vi "Dequeue Message.vi"(8 "error in (no error)":errorcluster, 10 "queue in":refnum<queue>) -> (0 "error out":errorcluster, 2 "queue out":refnum<queue>, 3 "Message out":refnum<class "Message.lvclass">)   [LabVIEW 2021, in "Architecture.lvlib" / "Message.lvclass"]
uses:
  Message.lvclass
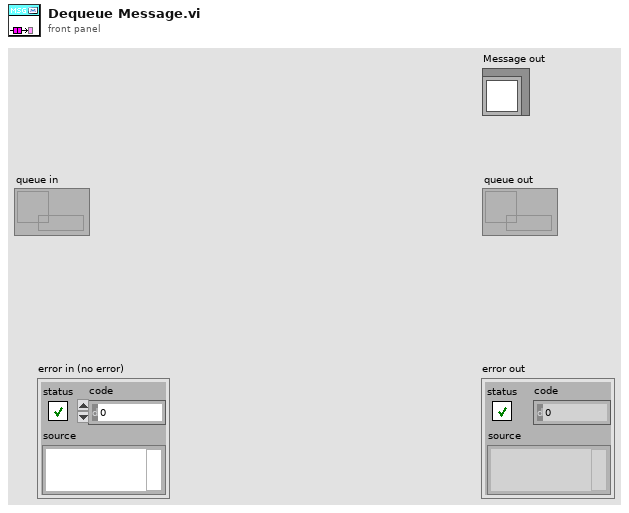
[diagram p1: front panel]
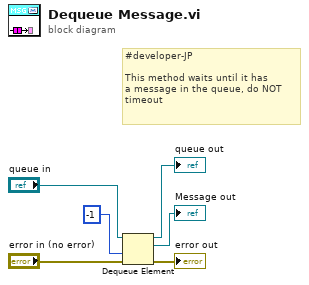
[diagram p0: block diagram]
diagram:
  # "#developer-JP\n\nThis method waits until it has \na message in the queue, do NOT \ntimeout"
  n1 = Dequeue Element(queue="queue in", timeout in ms (-1)=-1, error in (no error)="error in (no error)") -> (queue out=→"queue out":refnum<queue>, element=→"Message out":refnum<class "Message.lvclass">, error out=→"error out":errorcluster)  [unwired: 1 out]
